vi "Read Dimensions.vi"(8 "error in (no error)":errorcluster, 11 "Cube in":refnum<class "Cube.lvclass">) -> (0 "error out":errorcluster, 2 "Dimensions":T1, 3 "Cube out":refnum<class "Cube.lvclass">)   [LabVIEW 2019, in "22.lvlib" / "Cube.lvclass"]
uses:
  Cube.lvclass
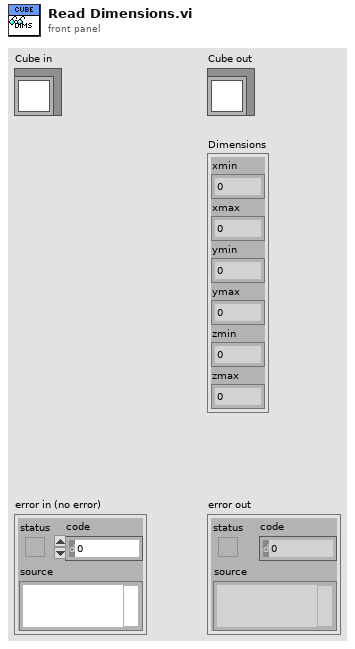
[diagram p1: front panel]
types:
  T1 = cluster{"xmin":i64, "xmax":i64, "ymin":i64, "ymax":i64, "zmin":i64, "zmax":i64}
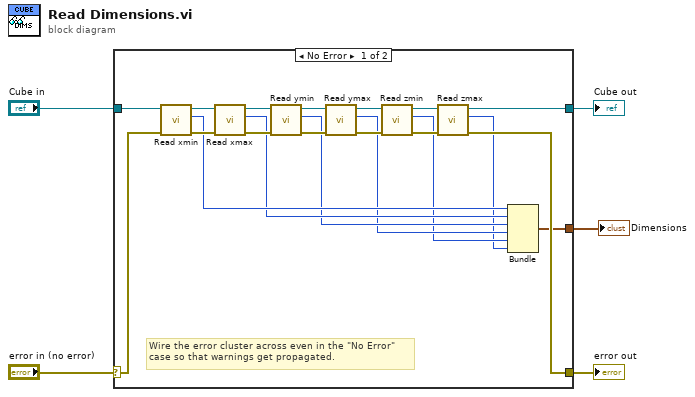
[diagram p0: block diagram]
diagram:
  n1 = case shown="No Error" "error in (no error)" {
    selector: "error in (no error)" -> [w14 w28]
    tunnel: [w13 w28] -> w4
    tunnel: [w15 w27] -> w2
    tunnel: "Cube in" -> [w16 w27]
    tunnel: [w6 _] -> w1
    frame No Error {
      # "Wire the error cluster across even in the \"No Error\"\ncase so that warnings get propagated."
      n2 = call-dynamic "Read xmin.vi"("error in (no error)"=w14, "Cube in"=w16) -> ("error out"=w18:errorcluster, "xmin"=w12:i64, "Cube out"=w17:refnum<class "Cube.lvclass">)  [unwired: 7 in]
      n3 = call-dynamic "Read xmax.vi"("error in (no error)"=w18, "Cube in"=w17) -> ("error out"=w20:errorcluster, "xmax"=w11:i64, "Cube out"=w19:refnum<class "Cube.lvclass">)  [unwired: 7 in]
      n4 = call-dynamic "Read ymin.vi"("error in (no error)"=w20, "Cube in"=w19) -> ("error out"=w22:errorcluster, "ymin"=w10:i64, "Cube out"=w21:refnum<class "Cube.lvclass">)  [unwired: 7 in]
      n5 = call-dynamic "Read ymax.vi"("error in (no error)"=w22, "Cube in"=w21) -> ("error out"=w24:errorcluster, "ymax"=w9:i64, "Cube out"=w23:refnum<class "Cube.lvclass">)  [unwired: 7 in]
      n6 = call-dynamic "Read zmin.vi"("error in (no error)"=w24, "Cube in"=w23) -> ("error out"=w26:errorcluster, "zmin"=w8:i64, "Cube out"=w25:refnum<class "Cube.lvclass">)  [unwired: 7 in]
      n7 = call-dynamic "Read zmax.vi"("error in (no error)"=w26, "Cube in"=w25) -> ("error out"=w13:errorcluster, "zmax"=w7:i64, "Cube out"=w15:refnum<class "Cube.lvclass">)  [unwired: 7 in]
      n8 = Bundle("xmin"=w12, "xmax"=w11, "ymin"=w10, "ymax"=w9, "zmin"=w8, "zmax"=w7) -> (w6:T1)  [unwired: 1 in]
    }
    frame Error {
    }
  }
  "error out" <- w4
  "Cube out" <- w2
  "Dimensions" <- w1
